vi "Basic ITC-Init.vi"(0 "Connection Details":T17={"VISA resource name"="", "Comms Layer"=enum."Ethernet TCP/IP", "IP Address"="", "Serial Configuration"={"Baud Rate"=115200, "Parity"=0, "Data Bits"=8, "Stop Bits"=10, "Flow Control"=0}, "ISOBUS address"=-1} {"Serial Configuration"."Flow Control" items=["None", "XON/XOFF", "RTS/CTS", "XON/XOFF & RTS/CTS", "DTR/DSR", "XON/XOFF & DTR/DSR"]; "Serial Configuration"."Stop Bits" items=["1.0"=10, "2.0"=20]; "Serial Configuration"."Data Bits" items=["7"=7, "8"=8]; "Serial Configuration"."Parity" items=["None", "Odd", "Even"]; "Serial Configuration"."Baud Rate" items=["300"=300, "600"=600, "1200"=1200, "2400"=2400, "4800"=4800, "9600"=9600, "14400"=14400, "19200"=19200, "38400"=38400, "57600"=57600, "115200"=115200]}, 7 "ID Query (True)":bool, 9 "Clear Previous Connections (False)":bool, 11 "error in (no error)":errorcluster) -> (3 "Device Details":T13, 4 "Merc Ref Out":T18, 6 "Device_ref_Array":T18[](array[typedef]), 8 "Ch_type_index":i32[](array[numeric]), 10 "Device_Present?":bool[](array[boolean]), 12 "ISOBUS address":T16=-1, 15 "error out":errorcluster)   [LabVIEW 2013, in "Mercury iXX.lvlib"]
uses:
  Mercury iXX.lvlib
  Public/Libraries/System/Read/DateTime (Read).vi
  Public/Libraries/System.lvlib
  Public/Libraries/System/Open/Open System.vi
  Public/Libraries/System/Read/Catalogue (Read).vi
  Public/Libraries/Level Meter/Open/Open Level Meter Device.vi
  Public/Libraries/Level Meter.lvlib
  Public/Libraries/Temperature/Open/Open Temperature Device.vi
  Public/Libraries/Temperature.lvlib
  Public/Libraries/Heater/Open/Open Heater Device.vi
  Public/Libraries/Heater.lvlib
  Public/Libraries/Auxiliary/Open/Open Auxiliary Device.vi
  Public/Libraries/Auxiliary.lvlib
  Public/Libraries/Pressure/Open/Open Pressure Device.vi
  Public/Libraries/Pressure.lvlib
  Public/Controls/Comms Transport Layer.ctl
  Private/Controls/Query Dynamic Reference.ctl
  Public/Controls/Mercury Reference.ctl
  Public/Libraries/Temperature/Configuration/Read/Temperature Device (Read).vi
  Public/Libraries/Heater/Configuration/Read/Heater Device (Read).vi
  Public/Libraries/Pressure/Configuration/Read/Serial Number (Read).vi
  Public/Libraries/Level Meter/Configuration/Read/Serial Number (Read).vi
  Public/Libraries/Auxiliary/Configuration/Read/Serial Number (Read).vi
  Public/Controls/Serial Settings.ctl
  Public/Controls/ISOBus Address.ctl
  Public/Libraries/Temperature/Controls/Loop Cluster.ctl
  Public/Controls/Manufacturing Data.ctl
  Public/Libraries/Temperature/Controls/Temperature Sensor Type.ctl
  Public/Libraries/Temperature/Controls/Excitation Type.ctl
  Public/Libraries/Temperature/Controls/Excitation Cluster.ctl
  Public/Libraries/Temperature/Controls/Calibration Interpolation.ctl
  Public/Libraries/Temperature/Controls/Calibration Cluster.ctl
  Public/Libraries/Temperature/Controls/Temperature Signals Cluster.ctl
  Public/Libraries/Temperature/Controls/Temperature Device (Read).ctl
  Public/Libraries/Heater/Controls/Heater Signals Cluster.ctl
  Public/Libraries/Heater/Controls/Heater Device (Read).ctl
panel:
  in  "Htr Dev Det":T1
  in  "Device Det":T4
  in  "Tab Control":T12(tab)
  out "Sys_time_stamp":timestamp
  out "Temp Dev Settings Array":T4[](array[typedef])
  out "Heater Device Settings Array":T1[](array[typedef])
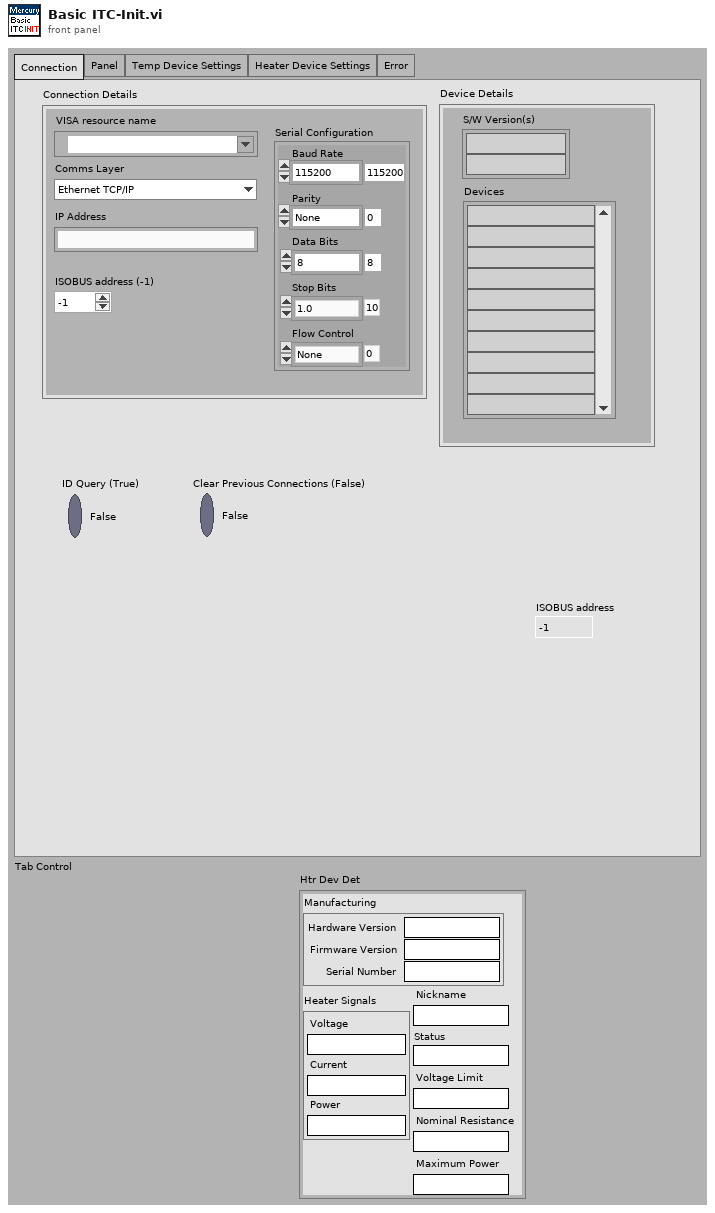
[diagram p1: front panel]
types:
  T1 = typedef "Mercury iXX.lvlib/Heater.lvlib/Heater Device (Read).ctl" = cluster{"Manufacturing":T2, "Nickname":string, "Voltage Limit":string, "Nominal Resistance":string, "Maximum Power":string, "Heater Signals":T3, "Status":string}
  T2 = typedef "Mercury iXX.lvlib/Manufacturing Data.ctl" = cluster{"Hardware Version":string, "Firmware Version":string, "Serial Number":string}
  T3 = typedef "Mercury iXX.lvlib/Heater.lvlib/Heater Signals Cluster.ctl" = cluster{"Voltage":string, "Current":string, "Power":string}
  T4 = typedef "Mercury iXX.lvlib/Temperature.lvlib/Temperature Device (Read).ctl" = cluster{"Manufacturing":T2, "Temperature Sensor Type":T5, "Excitation":T6, "Calibration":T8, "Control Loop":T10, "Temperature Signals":T11, "Nickname":string, "Status":string}
  T5 = typedef "Mercury iXX.lvlib/Temperature.lvlib/Temperature Sensor Type.ctl" = string
  T6 = typedef "Mercury iXX.lvlib/Temperature.lvlib/Excitation Cluster.ctl" = cluster{"Excitation Type":T7, "Magnitude":string}
  T7 = typedef "Mercury iXX.lvlib/Temperature.lvlib/Excitation Type.ctl" = string
  T8 = typedef "Mercury iXX.lvlib/Temperature.lvlib/Calibration Cluster.ctl" = cluster{"Filename":string, "Interpolation":T9, "Scaling Factor":string, "Offset Factor":string, "Hot Limit":string, "Cold Limit":string, "Last Calibration":string, "Reference":string}
  T9 = typedef "Mercury iXX.lvlib/Temperature.lvlib/Calibration Interpolation.ctl" = string
  T10 = typedef "Mercury iXX.lvlib/Temperature.lvlib/Loop Cluster.ctl" = cluster{"Heater":string, "Auxiliary":string, "Heater Auto":string, "Percentage Heat":string, "Temperature Set Point":string, "PID Auto (from file)":string, "P Value":string, "I Value":string, "D Value":string, "Auto PID Table Filename":string, "Flow Auto":string, "Target Heater Table":string, "Sweep mode":string, "Sweep Table Filename":string, "Percentage Flow":string}
  T11 = typedef "Mercury iXX.lvlib/Temperature.lvlib/Temperature Signals Cluster.ctl" = cluster{"Voltage":string, "Current":string, "Power":string, "Resistance":string, "Temperature":string, "Sensitivity":string, "Reference":string}
  T12 = enum32{"Connection", "Panel", "Temp Device Settings", "Heater Device Settings", "Error"}
  T13 = cluster{"Devices":string[], "S/W Version(s)":string[]}
  T14 = typedef "Mercury iXX.lvlib/Comms Transport Layer.ctl" = enum16{"Ethernet TCP/IP", "USB", "ISOBus - RS-232", "GPIB"}
  T15 = typedef "Mercury iXX.lvlib/Serial Settings.ctl" = cluster{"Baud Rate":u32, "Parity":u16, "Data Bits":u16, "Stop Bits":u16, "Flow Control":u16}
  T16 = typedef "Mercury iXX.lvlib/ISOBus Address.ctl" = i32
  T17 = cluster{"VISA resource name":refnum<visa-resource-name>, "Comms Layer":T14, "IP Address":string, "Serial Configuration":T15, "ISOBUS address":T16}
  T18 = typedef "Mercury iXX.lvlib/Mercury Reference.ctl" = cluster{"Comms":refnum<visa-resource-name>, "Device ID":string[], "Comms Layer":T14, "Command":string, "Query reference":T19}
  T19 = typedef "Mercury iXX.lvlib/Query Dynamic Reference.ctl" = refnum<vi>
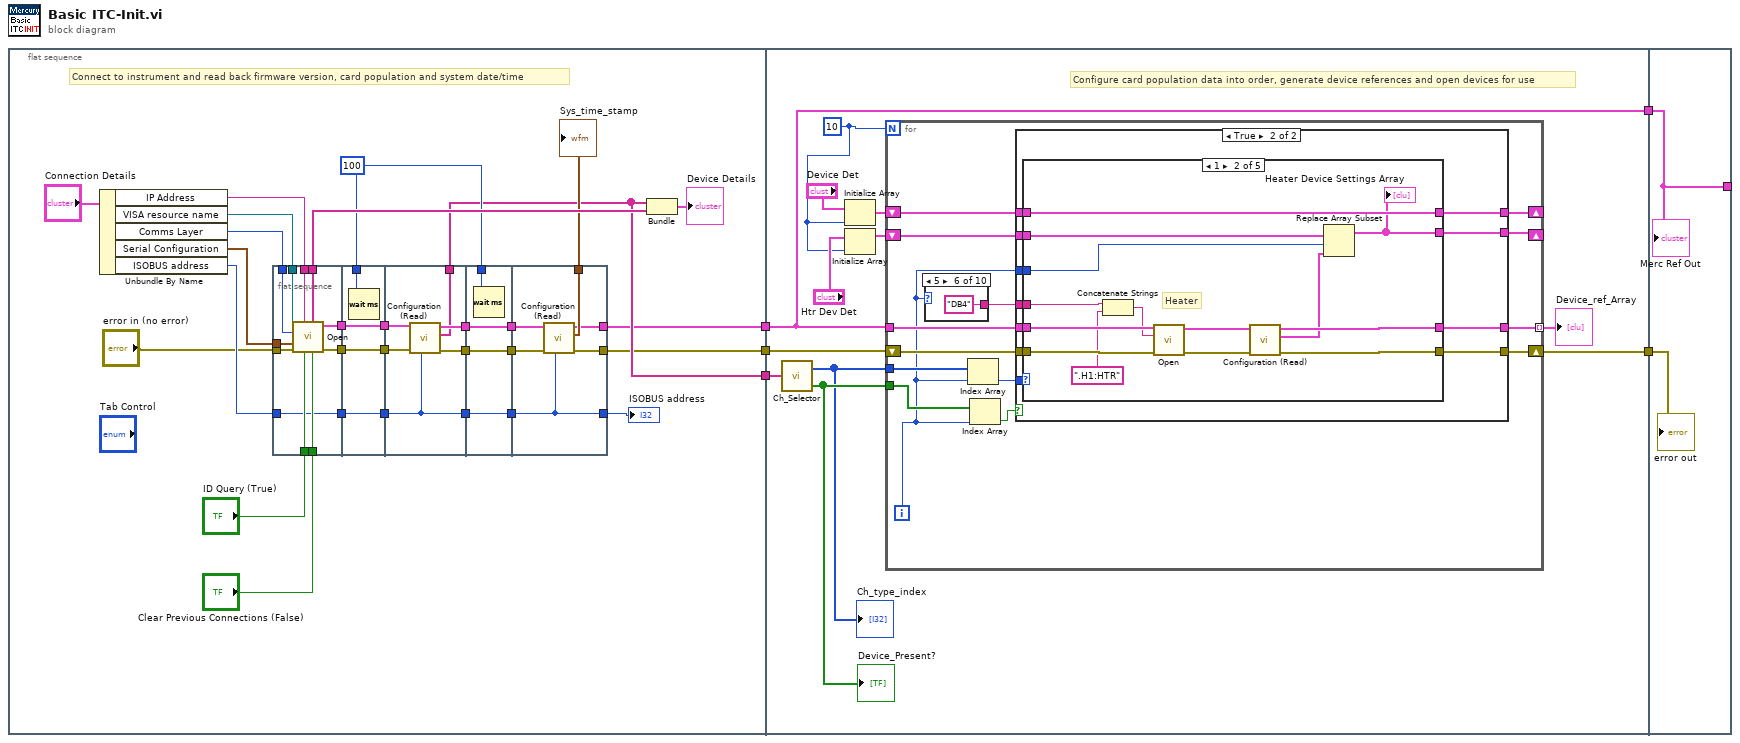
[diagram p0: block diagram]
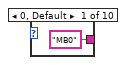
[diagram p2: hidden frame]
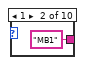
[diagram p3: hidden frame]
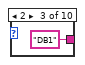
[diagram p4: hidden frame]
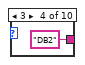
[diagram p5: hidden frame]
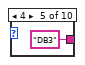
[diagram p6: hidden frame]
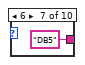
[diagram p7: hidden frame]
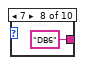
[diagram p8: hidden frame]
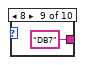
[diagram p9: hidden frame]
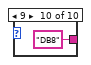
[diagram p10: hidden frame]
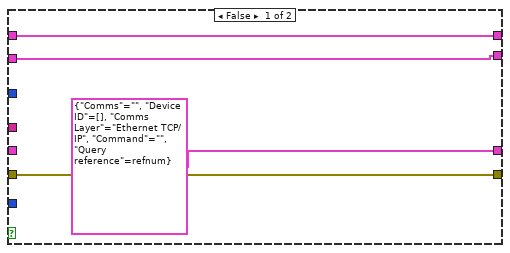
[diagram p11: hidden frame]
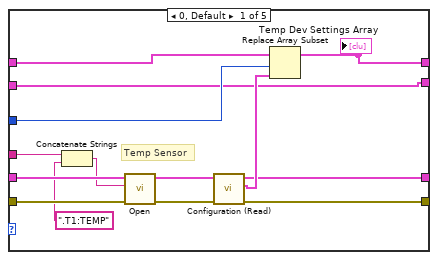
[diagram p12: hidden frame]
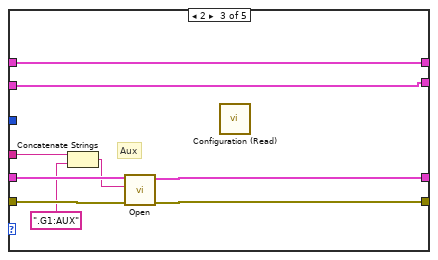
[diagram p13: hidden frame]
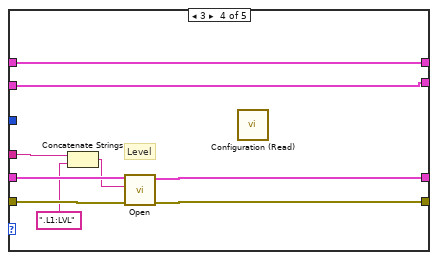
[diagram p14: hidden frame]
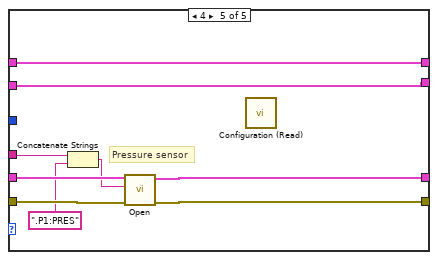
[diagram p15: hidden frame]
diagram:
  n1 = flat-sequence {
    tunnel: [w9] -> w5
    tunnel: [w8] -> w4
    tunnel: [w6] -> w3
    tunnel: w5 -> [w74]
    tunnel: w4 -> [w72]
    tunnel: w3 -> [w73]
    tunnel: [w72] -> w2
    tunnel: [w71] -> w1
    tunnel: w2 -> [w172]
    tunnel: w1 -> [w173]
    tunnel: [w172] -> _
    frame #0 {
      w12 = i16 100 ("Interval between messages (ms)")
      # "Connect to instrument and read back firmware version, card population and system date/time"
      n2 = Unbundle By Name("Connection Details") -> ("IP Address"=w18:string, "VISA resource name"=w17:refnum<visa-resource-name>, "Comms Layer"=w16:T14, "Serial Configuration"=w19:T15, "ISOBUS address"=w13:T16)
      n3 = flat-sequence {
        tunnel: "error in (no error)" -> [w45]
        tunnel: "ID Query (True)" -> [w44]
        tunnel: "Clear Previous Connections (False)" -> [w43]
        tunnel: w19 -> [w40]
        tunnel: w18 -> [w39]
        tunnel: w17 -> [w38]
        tunnel: w16 -> [w37]
        tunnel: [w36] -> w14
        tunnel: [w42] -> w34
        tunnel: [w41] -> w33
        tunnel: w13 -> [w35]
        tunnel: [w35] -> w32
        tunnel: w34 -> [w49]
        tunnel: w33 -> [w48]
        tunnel: [w49] -> w31
        tunnel: [w48] -> w30
        tunnel: w32 -> [w47]
        tunnel: [w47] -> w29
        tunnel: w12 -> [w46]
        tunnel: w31 -> [w54]
        tunnel: w30 -> [w53]
        tunnel: w29 -> [w55]
        tunnel: [w55] -> w28
        tunnel: [w52] -> w27
        tunnel: [w51] -> w26
        tunnel: [w50] -> w9
        tunnel: w28 -> [w59]
        tunnel: w27 -> [w58]
        tunnel: w26 -> [w57]
        tunnel: w12 -> [w56]
        tunnel: [w59] -> w25
        tunnel: [w58] -> w24
        tunnel: [w57] -> w23
        tunnel: w25 -> [w63]
        tunnel: w24 -> [w64]
        tunnel: w23 -> [w65]
        tunnel: [w62] -> w11
        tunnel: [w63] -> w7
        tunnel: [w61] -> w8
        tunnel: [w60] -> w6
        frame #0 {
          n4 = call-poly "Open.vi"("Clear Previous Connections (False)"=w43, "ID Query (True)"=w44, "IP Address"=w39, "error in (no error)"=w45, "Serial Configuration"=w40, "Comms Layer"=w37, "VISA resource name"=w38) -> ("error out"=w41:errorcluster, "Mercury Reference Out"=w42:T18, "S/W Version(s)"=w36:string[])  [unwired: 2 out]
        }
        frame #1 {
          n5 = Wait (ms)(milliseconds to wait=w46) -> ()  [unwired: 1 out]
        }
        frame #2 {
          n6 = call-poly "Configuration (Read).vi"("ISOBUS address"=w55, "error in"=w53, "Mercury Reference In"=w54) -> ("error out"=w52:errorcluster, "Devices"=w50:string[], "Mercury Reference Out"=w51:T18)  [unwired: 6 out]
        }
        frame #3 {
          n7 = Wait (ms)(milliseconds to wait=w56) -> ()  [unwired: 1 out]
        }
        frame #4 {
          n8 = call-poly "Configuration (Read).vi"("ISOBUS address"=w63, "error in"=w64, "Mercury Reference In"=w65) -> ("error out"=w60:errorcluster, "time stamp"=w62:timestamp, "Mercury Reference Out"=w61:T18)  [unwired: 6 out]
        }
      }
      n9 = Bundle("Devices"=w9, "S/W Version(s)"=w14) -> (→"Device Details":T13)  [unwired: 1 out]
      "Sys_time_stamp" <- w11
      "ISOBUS address" <- w7
    }
    frame #1 {
      w67 = 10
      # "Configure card population data into order, generate device references and open devices for use"
      n10 = call "Ch_Selector.vi"("Devices"=w74) -> ("Ch_type_index"=w76:i32[], "Device_Present?"=w77:bool[])
      "Ch_type_index" <- w76
      "Device_Present?" <- w77
      n11 = Initialize Array("Device Det", w67) -> (w69:T4[])
      n12 = Initialize Array("Htr Dev Det", w67) -> (w66:T1[])
      n13 = for {
        N: w67 -> [_]
        tunnel: w72 -> [w91]
        tunnel: [w90] -> w75 mode=indexing
        tunnel: w76 -> [w89]
        tunnel: w77 -> [w88]
        shift-right: [w83] -> w71
        shift-left: w73 -> [w84]
        shift-right: [w81] -> _
        shift-left: w69 -> [w80]
        shift-right: [w79] -> _
        shift-left: w66 -> [w78]
        i -> [w82]
        n14 = case shown="5" w82 {
          tunnel: ["MB0" "MB1" "DB1" "DB2" "DB3" "DB4" "DB5" "DB6" "DB7" "DB8"] -> w85
          frame 0, Default {
          }
          frame 1 {
          }
          frame 2 {
          }
          frame 3 {
          }
          frame 4 {
          }
          frame 5 {
          }
          frame 6 {
          }
          frame 7 {
          }
          frame 8 {
          }
          frame 9 {
          }
        }
        n15 = Index Array(array=w89, index=w82) -> (element=w86:i32)
        n16 = Index Array(array=w88, index=w82) -> (element=w87:bool)
        n17 = case shown="True" w87 {
          tunnel: w91 -> [_ w116]
          tunnel: w84 -> [w104 w115]
          tunnel: [T18 {"Comms"="", "Device ID"=[], "Comms Layer"=enum."Ethernet TCP/IP", "Command"="", "Query reference"=refnum} ("Mercury Reference Out") w114] -> w90
          tunnel: [w104 w113] -> w83
          tunnel: w86 -> [_ w112]
          tunnel: w85 -> [_ w111]
          tunnel: w82 -> [_ w110]
          tunnel: [w103 w108] -> w81
          tunnel: w80 -> [w103 w109]
          tunnel: [w102 w107] -> w79
          tunnel: w78 -> [w102 w106]
          frame False {
          }
          frame True {
            n18 = case shown="1" w112 {
              tunnel: w115 -> [w130 w144 w153 w162 w171]
              tunnel: w116 -> [w129 w143 w152 w161 w170]
              tunnel: [w120 w137 w151 w160 w169] -> w114
              tunnel: [w119 w136 w150 w159 w168] -> w113
              tunnel: w111 -> [w128 w140 w147 w156 w165]
              tunnel: w110 -> [w123 w135 _ _ _]
              tunnel: [w118 w133 w146 w155 w164] -> w108
              tunnel: w109 -> [w121 w133 w146 w155 w164]
              tunnel: [w117 w131 w145 w154 w163] -> w107
              tunnel: w106 -> [w117 w132 w145 w154 w163]
              frame 0, Default {
                # "Temp Sensor"
                n19 = Concatenate Strings(w128, ".T1:TEMP" ("Device Identifier")) -> (w126:string)
                n20 = call-poly "Open.vi"("error in (no error)"=w130, "Device Identifier"=w126, "Mercury Reference In"=w129) -> ("error out"=w125:errorcluster, "Mercury Reference Out"=w124:T18)  [unwired: 1 in, 6 out]
                n21 = call-poly "Configuration (Read).vi"("error in"=w125, "Mercury Reference In"=w124) -> ("error out"=w119:errorcluster, "Device Details"=w122:T4, "Mercury Reference Out"=w120:T18)  [unwired: 1 in, 6 out]
                n22 = Replace Array Subset(array=w121, new element=w122, index=w123) -> (w118:T4[])
                "Temp Dev Settings Array" <- w118
              }
              frame 1 {
                # "Heater"
                n23 = Concatenate Strings(w140, ".H1:HTR" ("Device Identifier")) -> (w141:string)
                n24 = call-poly "Open.vi"("error in (no error)"=w144, "Device Identifier"=w141, "Mercury Reference In"=w143) -> ("error out"=w139:errorcluster, "Mercury Reference Out"=w138:T18)  [unwired: 7 in]
                n25 = call-poly "Configuration (Read).vi"("error in"=w139, "Mercury Reference In"=w138) -> ("error out"=w136:errorcluster, "Device Details"=w134:T1, "Mercury Reference Out"=w137:T18)  [unwired: 1 in, 6 out]
                n26 = Replace Array Subset(array=w132, new element=w134, index=w135) -> (w131:T1[])
                "Heater Device Settings Array" <- w131
              }
              frame 2 {
                # "Aux"
                n27 = Concatenate Strings(w147, ".G1:AUX" ("Device Identifier")) -> (w148:string)
                n28 = call-poly "Open.vi"("error in (no error)"=w153, "Device Identifier"=w148, "Mercury Reference In"=w152) -> ("error out"=w150:errorcluster, "Mercury Reference Out"=w151:T18)  [unwired: 7 out]
                n29 = call-poly "Configuration (Read).vi"() -> ()  [unwired: 8 in, 4 out]
              }
              frame 3 {
                # "Level"
                n30 = Concatenate Strings(w156, ".L1:LVL" ("Device Identifier")) -> (w157:string)
                n31 = call-poly "Open.vi"("error in (no error)"=w162, "Device Identifier"=w157, "Mercury Reference In"=w161) -> ("error out"=w159:errorcluster, "Mercury Reference Out"=w160:T18)  [unwired: 7 out]
                n32 = call-poly "Configuration (Read).vi"() -> ()  [unwired: 8 in, 4 out]
              }
              frame 4 {
                # "Pressure sensor"
                n33 = Concatenate Strings(w165, ".P1:PRES" ("Device Identifier")) -> (w166:string)
                n34 = call-poly "Open.vi"("error in (no error)"=w171, "Device Identifier"=w166, "Mercury Reference In"=w170) -> ("error out"=w168:errorcluster, "Mercury Reference Out"=w169:T18)  [unwired: 7 out]
                n35 = call-poly "Configuration (Read).vi"() -> ()  [unwired: 8 in, 4 out]
              }
            }
          }
        }
      }
      "Device_ref_Array" <- w75
    }
    frame #2 {
      "error out" <- w173
      "Merc Ref Out" <- w172
    }
  }
